vi "Inverse Fast Hilbert Transform PtByPt.vi"(2 "initialize":bool, 3 "sample length":i32=100, 5 "x":dbl format="%0.2f") -> (0 "error":i32, 1 "Inverse Hilbert{X}":dbl[](array[numeric]))   [LabVIEW 2020, in "NI_PtbyPt.lvlib"]
doc: "Computes the inverse fast Hilbert transform of the set of input data points specified by <B>sample length</B> using Fourier transform identities."
uses:
  <vilib>/ptbypt/NI_PtbyPt.lvlib
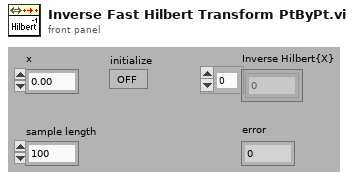
[diagram p1: front panel]
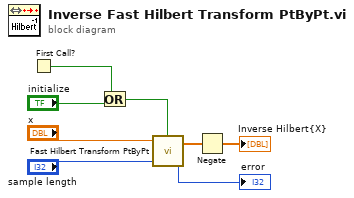
[diagram p0: block diagram]
diagram:
  n1 = First Call?() -> (First Call?: T/F=w1:bool)
  n2 = Or(x=w1, y="initialize") -> (x .or. y?=w2:bool)
  n3 = call <vilib>:"Fast Hilbert Transform PtByPt.vi"("initialize"=w2, "sample length"="sample length", "x"="x") -> ("error"=→"error":i32, "Hilbert{X}"=w6:dbl[])  [unwired: 1 in]
  n4 = Negate(x=w6) -> (-x=→"Inverse Hilbert{X}":dbl[])
